vi "filter.configuration.vi"(10 "Cluster":T17, 11 "filter.data in":T1 {"get.state"."v"."Quantity" format="%.0x"; "get.state"."v"."OrderId" format="%.0x"; "mem.cmd"."ord.2"."v"."Quantity" format="%016x"; "mem.cmd"."ord.2"."v"."OrderId" format="%016x"; "mem.cmd"."ord.1"."v"."Quantity" format="%016x"; "mem.cmd"."ord.1"."v"."OrderId" format="%016x"; "mem.cmd"."ticker"."v"."Symbol" format="%016x"; "mem.cmd"."order.slot.value"."Quantity" format="%016x"; "mem.cmd"."order.slot.value"."OrderId" format="%016x"; "debug"."v"."slot.3" format="%.0x"; "debug"."v"."slot.2" format="%.0x"; "debug"."v"."slot.1" format="%.0x"; "debug"."v"."slot.0" format="%.0x"; "Scratch"."OrderId" format="%016x"; "hash.2"."data.in" format="%.0x"; "hash.2"."crc32.out" format="%.0x"; "hash.1"."data.in" format="%.0x"; "hash.1"."crc32.out" format="%.0x"}) -> (2 "Boolean":bool, 3 "filter.data out":T1 {"get.state"."v"."Quantity" format="%.0x"; "get.state"."v"."OrderId" format="%.0x"; "mem.cmd"."ord.2"."v"."Quantity" format="%016x"; "mem.cmd"."ord.2"."v"."OrderId" format="%016x"; "mem.cmd"."ord.1"."v"."Quantity" format="%016x"; "mem.cmd"."ord.1"."v"."OrderId" format="%016x"; "mem.cmd"."ticker"."v"."Symbol" format="%016x"; "mem.cmd"."order.slot.value"."Quantity" format="%016x"; "mem.cmd"."order.slot.value"."OrderId" format="%016x"; "debug"."v"."slot.3" format="%.0x"; "debug"."v"."slot.2" format="%.0x"; "debug"."v"."slot.1" format="%.0x"; "debug"."v"."slot.0" format="%.0x"; "Scratch"."OrderId" format="%016x"; "hash.2"."data.in" format="%.0x"; "hash.2"."crc32.out" format="%.0x"; "hash.1"."data.in" format="%.0x"; "hash.1"."crc32.out" format="%.0x"})   [LabVIEW 2020]
uses:
  order.slot.ctl
  ticker.slot.ctl
  filter.memory.command.ctl
  filter.states.ctl
  order.slot.hm.ctl
  order.slot.access.ctl
  ticker.slot.access.ctl
  filter.debug.slot.ctl
  filter.debug.ctl
  filter.data.scratch.ctl
  Market.Data.Common/fpga/orderbook.command.ctl
  Market.Data.Common/fpga/fpganow.common.fpga.lvlib
  filter.data.ctl
  filter.state.slot.ctl
  filter.state.ctl
  Market.Data.Common/fpga/orderbook.command.type.ctl
  filter.hash.ctl
  Filter.lvclass
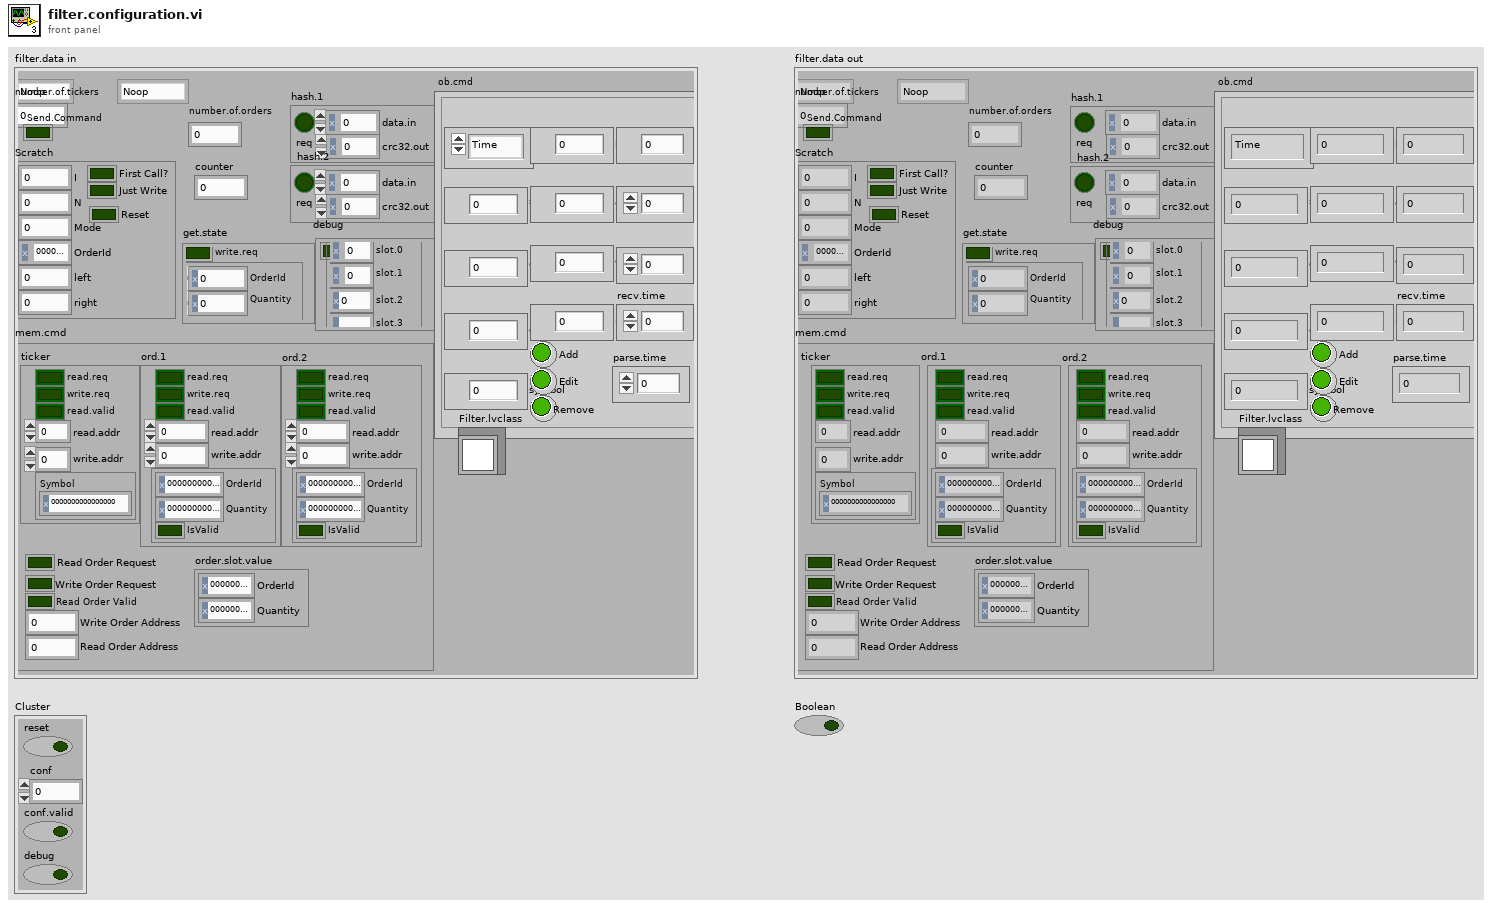
[diagram p1: front panel]
types:
  T1 = typedef "filter.data.ctl" = cluster{"filter.state":T2, "number.of.tickers":u32, "filter.saved.state":T2, "Send.Command":bool, "hash.1":T3, "hash.2":T3, "Scratch":T4, "debug":T5, "mem.cmd":T7, "get.state":T13, "ob.cmd":T15, "number.of.orders":u32, "Filter.lvclass":refnum<class "Filter.lvclass">, "counter":i16}
  T2 = typedef "filter.states.ctl" = enum16{"Noop", "Reset", "Debug", "Configuration", "Wait.for.Command", "Filter.Add", "Filter.Other", "Insert.Order", "Delete Order", "Get.State", "Get.Watchlist", "Get.Memory"}
  T3 = typedef "filter.hash.ctl" = cluster{"req":bool, "data.in":u64, "crc32.out":u32}
  T4 = typedef "filter.data.scratch.ctl" = cluster{"I":u32, "N":u32, "Mode":u32, "OrderId":u64, "First Call?":bool, "Just Write":bool, "left":u32, "right":u32, "Reset":bool}
  T5 = typedef "filter.debug.ctl" = cluster{"write":bool, "v":T6}
  T6 = typedef "filter.debug.slot.ctl" = cluster{"slot.0":u64, "slot.1":u64, "slot.2":u64, "slot.3":u64}
  T7 = typedef "filter.memory.command.ctl" = cluster{"Read Order Request":bool, "Write Order Request":bool, "Read Order Valid":bool, "Write Order Address":u32, "Read Order Address":u32, "order.slot.value":T8, "ticker":T9, "ord.1":T11, "ord.2":T11}
  T8 = typedef "order.slot.ctl" = cluster{"OrderId":u64, "Quantity":u64}
  T9 = typedef "ticker.slot.access.ctl" = cluster{"read.req":bool, "write.req":bool, "read.valid":bool, "read.addr":u32, "write.addr":u32, "v":T10}
  T10 = typedef "ticker.slot.ctl" = cluster{"Symbol":u64}
  T11 = typedef "order.slot.access.ctl" = cluster{"read.req":bool, "write.req":bool, "read.valid":bool, "read.addr":u32, "write.addr":u32, "v":T12}
  T12 = typedef "order.slot.hm.ctl" = cluster{"OrderId":u64, "Quantity":u64, "IsValid":bool}
  T13 = typedef "filter.state.ctl" = cluster{"write.req":bool, "v":T14}
  T14 = typedef "filter.state.slot.ctl" = cluster{"OrderId":u64, "Quantity":u64}
  T15 = typedef "fpganow.common.fpga.lvlib/orderbook.command.ctl" = cluster{"type":T16, "side":u8, "orderId ":u64, "quantity":u32, "symbol":u64, "price":u64, "executed.qty":u32, "canceled.qty":u32, "remaining.qty":u32, "seconds":u64, "nanoseconds":u64, "Add":bool, "Edit":bool, "Remove":bool, "seq no":u32, "recv.time":u64, "parse.time":u64}
  T16 = typedef "fpganow.common.fpga.lvlib/orderbook.command.type.ctl" = enum8{"Time", "AddOrder", "OrderExecuted", "OrderExecutedAtPrice", "ReduceSize", "ModifyOrder", "DeleteOrder", "Get.Everything", "Get.All.Orders", "Get.Top"}
  T17 = cluster{"reset":bool, "conf":u64, "conf.valid":bool, "debug":bool}
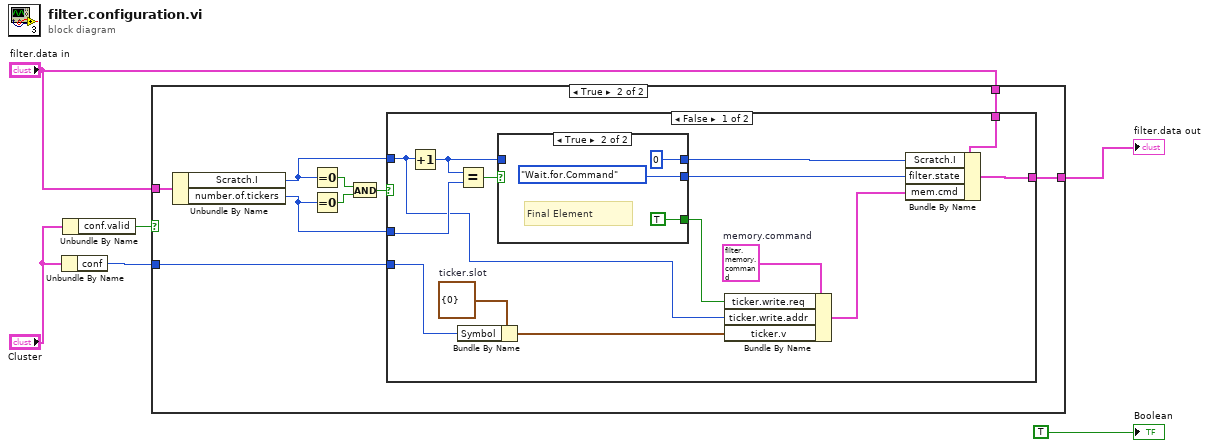
[diagram p0: block diagram]
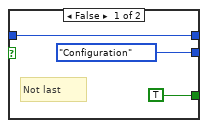
[diagram p3: hidden frame]
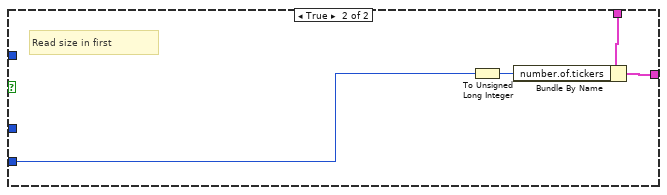
[diagram p4: hidden frame]
diagram:
  n1 = Unbundle By Name("Cluster") -> ("conf"=w5:u64)
  n2 = Unbundle By Name("Cluster") -> ("conf.valid"=w1:bool)
  n3 = case shown="True" w1 {
    tunnel: [w7 w12] -> w2
    tunnel: "filter.data in" -> [w7 w11]
    tunnel: "filter.data in" -> [_ w16]
    tunnel: w5 -> [_ w10]
    frame False {
      # "Noop"
    }
    frame True {
      n4 = Unbundle By Name(w16) -> ("Scratch.I"=w9:u32, "number.of.tickers"=w8:u32)
      n5 = Equal To 0?(x=w9) -> (x = 0?=w15:bool)
      n6 = Equal To 0?(x=w8) -> (x = 0?=w14:bool)
      n7 = And(x=w15, y=w14) -> (x .and. y?=w13:bool)
      n8 = case shown="False" w13 {
        tunnel: [w27 w37] -> w12
        tunnel: w11 -> [w28 w39]
        tunnel: w10 -> [w20 w40]
        tunnel: w9 -> [w18 _]
        tunnel: w8 -> [w30 _]
        frame False {
          w23 = T10 {"Symbol"=0}  # ticker.slot
          w24 = T7 {"Read Order Request"=FALSE, "Write Order Request"=FALSE, "Read Order Valid"=FALSE, "Write Order Address"=0, "Read Order Address"=0, "order.slot.value"={"OrderId"=0, "Quantity"=0}, "ticker"={"read.req"=FALSE, "write.req"=FALSE, "read.valid"=FALSE, "read.addr"=0, "write.addr"=0, "v"={"Symbol"=0}}, "ord.1"={"read.req"=FALSE, "write.req"=FALSE, "read.valid"=FALSE, "read.addr"=0, "write.addr"=0, "v"={"OrderId"=0, "Quantity"=0, "IsValid"=FALSE}}, "ord.2"={"read.req"=FALSE, "write.req"=FALSE, "read.valid"=FALSE, "read.addr"=0, "write.addr"=0, "v"={"OrderId"=0, "Quantity"=0, "IsValid"=FALSE}}}  # memory.command
          n9 = Increment(x=w18) -> (x+1=w25:u32)
          n10 = Equal?(x=w25, y=w30) -> (x = y?=w29:bool)
          n11 = Bundle By Name(cluster=w23, "Symbol"=w20) -> (w22:T10)
          n12 = case shown="True" w29 {
            tunnel: w25 -> [w32 _]
            tunnel: [w32 u32 0] -> w26
            tunnel: [filter.states."Configuration" ("filter.states") filter.states."Wait.for.Command" ("filter.states")] -> w19
            tunnel: [TRUE ("Write Order\nRequest") TRUE ("Write Order\nRequest")] -> w17
            frame False {
              # "Not last"
            }
            frame True {
              # "Final Element"
            }
          }
          n13 = Bundle By Name(cluster=w24, "ticker.write.req"=w17, "ticker.write.addr"=w18, "ticker.v"=w22) -> (w21:T7)
          n14 = Bundle By Name(cluster=w28, "Scratch.I"=w26, "filter.state"=w19, "mem.cmd"=w21) -> (w27:T1)
        }
        frame True {
          # "Read size in first"
          n15 = To Unsigned Long Integer(number=w40) -> (unsigned 32bit integer=w38:u32)
          n16 = Bundle By Name(cluster=w39, "number.of.tickers"=w38) -> (w37:T1)
        }
      }
    }
  }
  "filter.data out" <- w2
  "Boolean" <- TRUE
